vi "Read.vi"(11 "SeqLoaded Condition Config in":refnum<class "SeqLoaded Condition Config.lvclass">) -> (3 "Sequence":string)   [LabVIEW 2020, in "VolatusSeqConfig.lvlib" / "SeqLoaded Condition Config.lvclass"]
uses:
  SeqLoaded Condition Config.lvclass
  SeqLoaded Condition Config.lvclass/SeqLoaded Condition Config.ctl
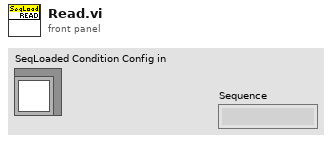
[diagram p1: front panel]
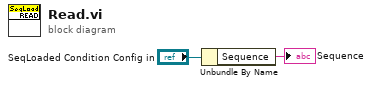
[diagram p0: block diagram]
diagram:
  n1 = Unbundle By Name("SeqLoaded Condition Config in") -> ("Sequence"=→"Sequence":string)
